vi "Destroy Transceiver Interface.vi"(8 "error in (no error)":errorcluster, 11 "Transceiver Interface in":refnum<class "Transceiver Interface.lvclass">) -> (0 "error out":errorcluster)   [LabVIEW 2017, in "Data Sharing Framework Engine.lvlib" / "Transceiver Interface.lvclass"]
uses:
  Transceiver Interface.lvclass
  C:/github/data-sharing-framework/Source/Data Sharing Framework Core/Engine/Interfaces/Engine Interface/Engine Interface.lvclass
  Engine Interface/Engine Interface.lvclass
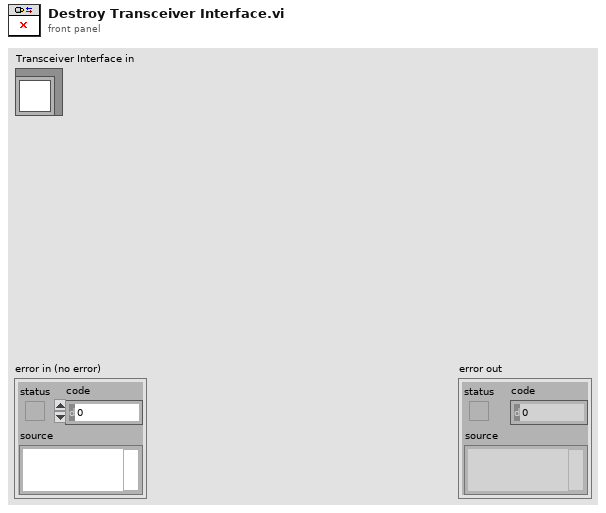
[diagram p1: front panel]
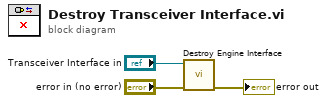
[diagram p0: block diagram]
diagram:
  n1 = call "Destroy Engine Interface.vi"("error in (no error)"="error in (no error)", "Interface in"="Transceiver Interface in") -> ("error out"=→"error out":errorcluster)  [unwired: 7 in, 2 out]
